vi "Lvi Write U32Data Pt.vi"(8 "error in (no error)":errorcluster, 9 "DataBuf":u32, 10 "timeout":dbl, 11 "TaskRef":i32) -> (0 "error out":errorcluster, 2 "function return":i32, 3 "TaskRef out":i32)   [LabVIEW 2022 SP3, in "DtLvLink.lvlib"]
doc: "Calls directly into the entry points of the DLL of the Data Acq SDK to write a data point from the specified task as an unsigned 32-bit integer."
uses:
  DtLvLink.lvlib
  <userlib>/LV-Link3/DtLvLink_64.dll
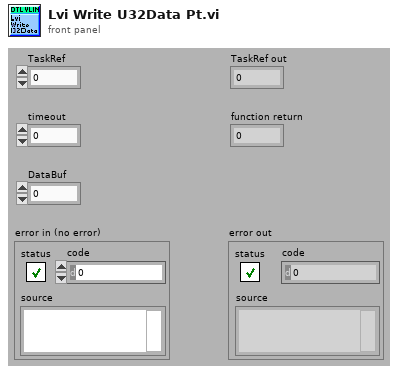
[diagram p1: front panel]
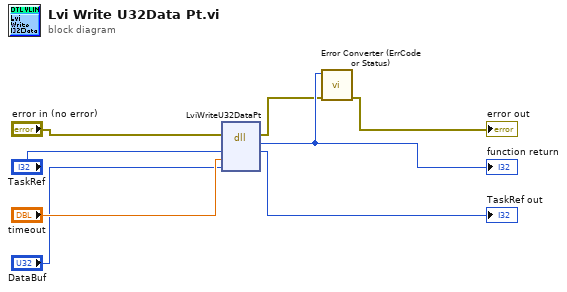
[diagram p0: block diagram]
diagram:
  n1 = dll-call lib="C:/Program Files/National Instruments/LabVIEW 2022/user.lib/LV-Link3/DtLvLink_64.*" fn="LviWriteU32DataPt"(error in="error in (no error)", "TaskRef"="TaskRef", "timeout"="timeout", "DataBuf"="DataBuf") -> (error out=w2:errorcluster, "return type"=w8:i32, "TaskRef"=→"TaskRef out":i32)  [unwired: 4 in, 1 out]
  "function return" <- w8
  n2 = call "Error Converter (ErrCode or Status).vi"("error in (no error)"=w2, "error code"=w8) -> ("error out"=→"error out":errorcluster)  [unwired: 9 in]
